vi "EXT.vi"(4 "Value":ext) -> (1 "Constant":refnum<class "Abs_Extended Float.lvclass">)   [LabVIEW 2021, in "Const_EXT.lvclass"]
uses:
  Const_EXT.lvclass
  Abs_Types/Extended Float/Abs_Extended Float.lvclass
  C:/Program Files (x86)/National Instruments/LabVIEW 2021/vi.lib/TSA/Abstract Data Classes/Abs_Types/Extended Float/Abs_Extended Float.lvclass
  Const_EXT.lvclass/Const_EXT.ctl
  Properties/Write Value.vi
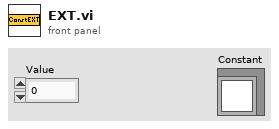
[diagram p1: front panel]
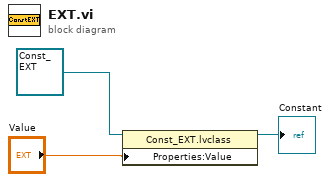
[diagram p0: block diagram]
diagram:
  n1 = property class="Const_EXT.lvclass"(reference=refnum<class "Const_EXT.lvclass"> refnum ("Constants.lvlib:Numeric.lvclass"), "Properties:Value"="Value") -> (reference out=→"Constant":refnum<class "Const_EXT.lvclass">)  [unwired: 1 in, 1 out]
